vi "MusicNotesGenerator.vi"() -> ()   [LabVIEW 2015]
uses:
  <vilib>/sound2/lvsound2.llb/Sound Output Write (DBL Single).vi
  <vilib>/measure/NI_MABase.lvlib
panel:
  in  "OK Button 12":bool
  in  "OK Button 11":bool
  in  "OK Button 10":bool
  in  "OK Button 9":bool
  in  "OK Button 8":bool
  in  "OK Button 7":bool
  in  "OK Button 6":bool
  in  "OK Button 5":bool
  in  "OK Button 4":bool
  in  "OK Button 3":bool
  in  "OK Button 2":bool
  in  "OK Button":bool
  in  "amplitude":dbl(knob)=5.0 scale=0.0..10.0
  out "Waveform Graph":waveform(dbl)(graph)={"t0"=timestamp(1457.0 s since 1904-01-01), "dt"=0.001, "Y"=array[1000 elements]}
  out "Waveform Chart":waveform(dbl)(graph)={"t0"=timestamp(1457.0 s since 1904-01-01), "dt"=0.001, "Y"=array[1000 elements]}
  in  "stop":bool
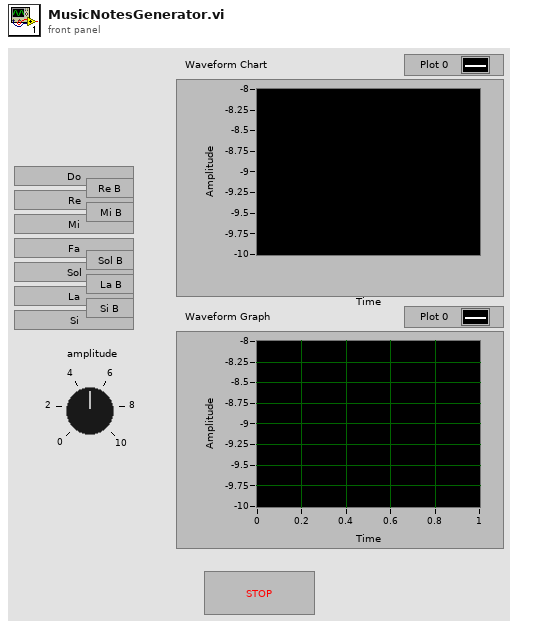
[diagram p1: front panel]
types:
  T1 = typedef "Sound Output Task ID.ctl" = u32
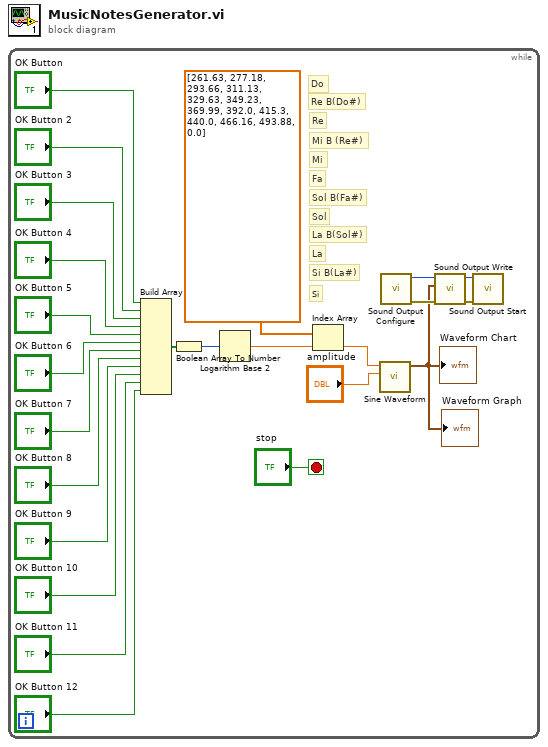
[diagram p0: block diagram]
diagram:
  n1 = while {
    stop <- "stop" stop-if-true
    # "Si"
    # "Si B(La#)"
    # "La"
    # "La B(Sol#)"
    # "Sol"
    # "Sol B(Fa#)"
    # "Fa"
    # "Mi"
    # "Mi B (Re#)"
    # "Re"
    # "Re B(Do#)"
    # "Do"
    n2 = Build Array("OK Button", "OK Button 2", "OK Button 3", "OK Button 4", "OK Button 5", "OK Button 6", "OK Button 7", "OK Button 8", "OK Button 9", "OK Button 10", "OK Button 11", "OK Button 12") -> (w11:bool[])
    n3 = Boolean Array To Number(Boolean array=w11) -> (number=w10:u32)
    n4 = Logarithm Base 2(1:w10) -> (0:w9:dbl)
    n5 = Index Array(array=dbl[] [261.63, 277.18, 293.66, 311.13, 329.63, 349.23, 369.99, 392.0, 415.3, 440.0, 466.16, 493.88, 0.0], index=w9) -> (element=w1:dbl)
    n6 = call <vilib>:"Sine Waveform.vi"("amplitude"="amplitude", "frequency"=w1) -> ("signal out"=w3:waveform(dbl))  [unwired: 8 in, 1 out]
    "Waveform Chart" <- w3
    "Waveform Graph" <- w3
    n7 = call <vilib>:"Sound Output Configure.vi"() -> ("error out"=w8:errorcluster, "task ID"=w7:T1)  [unwired: 10 in]
    n8 = call-poly <vilib>:"Sound Output Write.vi"("error in (no error)"=w8, "data"=w3, "task ID"=w7) -> ("error out"=w6:errorcluster, "task ID out"=w5:T1)  [unwired: 7 in]
    n9 = call <vilib>:"Sound Output Start.vi"("error in (no error)"=w6, "task ID"=w5) -> ()  [unwired: 8 in, 2 out]
  }
